vi "Write VI path.vi"(8 "error in":errorcluster, 10 "VI path":path, 11 "UI Reference configuration in":refnum<class "UI Reference configuration.lvclass">) -> (0 "error out":errorcluster, 3 "UI Reference configuration out":refnum<class "UI Reference configuration.lvclass">)   [LabVIEW 2013, in "UI Reference configuration.lvclass"]
uses:
  UI Reference configuration.lvclass
  UI Reference configuration.lvclass/UI Reference configuration.ctl
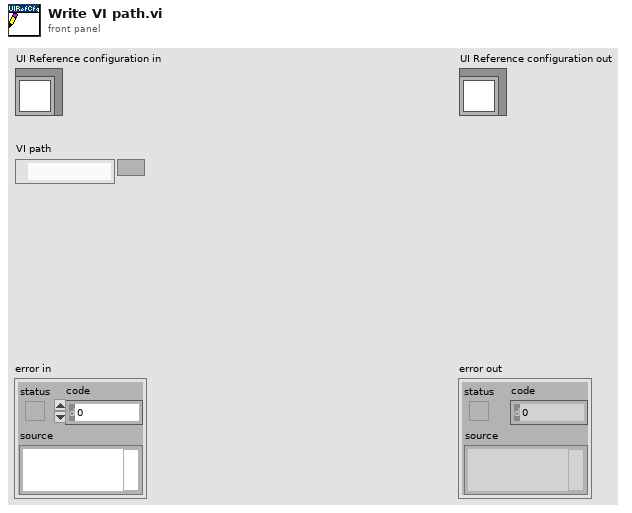
[diagram p1: front panel]
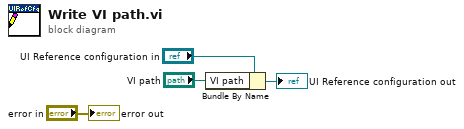
[diagram p0: block diagram]
diagram:
  n1 = Bundle By Name(cluster="UI Reference configuration in", "VI path"="VI path") -> (→"UI Reference configuration out":refnum<class "UI Reference configuration.lvclass">)
  "error out" <- "error in"
